vi "Release.vi"(8 "error in (no error)":errorcluster, 11 "Get Refnum in":refnum<class "Get Refnum.lvclass">) -> (0 "error out":errorcluster)   [LabVIEW 2020, in "Msg.lvlib" / "Get Refnum.lvclass"]
doc: "Release the queue reference and set the occurance to terminate the Data Access execution."
uses:
  Get Refnum.lvclass
  Get Refnum.lvclass/Get Refnum.ctl
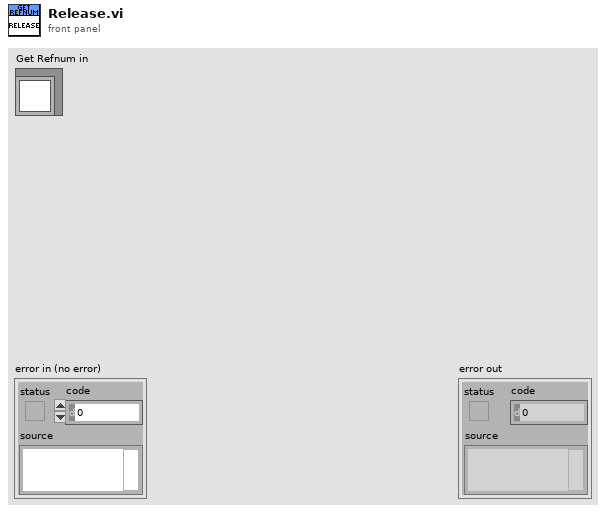
[diagram p1: front panel]
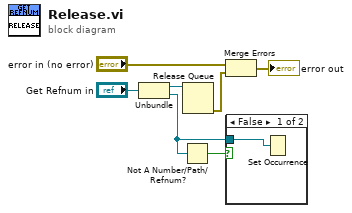
[diagram p0: block diagram]
diagram:
  n1 = Unbundle("Get Refnum in") -> (w5:refnum<queue>, w2:refnum<k4>)
  n2 = Not A Number/Path/Refnum?(number/path/refnum=w2) -> (NaN/Path/Refnum?=w1:bool)
  n3 = Release Queue(queue=w5) -> (error out=w3:errorcluster)  [unwired: 2 in, 2 out]
  n4 = Merge Errors("error in (no error)", w3) -> (→"error out":errorcluster)
  n5 = case shown="False" w1 {
    tunnel: w2 -> [w8 _]
    frame False {
      n6 = Set Occurrence(w8) -> ()
    }
    frame True {
    }
  }
